vi "FloatToHex.vi"(11 "浮点数":sgl[](array[numeric])) -> (3 "DCBA整形输出":u16[](array[numeric]) format="%04xH")   [LabVIEW 2016, in "斯坦道总磷总氮V2.lvlib"]
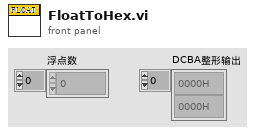
[diagram p1: front panel]
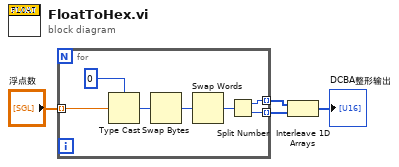
[diagram p0: block diagram]
diagram:
  n1 = for {
    tunnel: "浮点数" -> [w9] mode=indexing
    tunnel: [w8] -> w2 mode=indexing
    tunnel: [w7] -> w3 mode=indexing
    n2 = Type Cast(type=0, x=w9) -> (*(type *) &x=w6:i32)
    n3 = Swap Bytes(anything=w6) -> (byte swapped=w5:i32)
    n4 = Swap Words(1:w5) -> (0:w11:i32)
    n5 = Split Number(x=w11) -> (hi(x)=w8:u16, lo(x)=w7:u16)
  }
  n6 = Interleave 1D Arrays(w2, w3) -> (→"DCBA整形输出":u16[])
